vi "NI VeriStand - Open Workspace Tool.vi"(7 "Workspace Tool Path":path, 8 "error in (no error)":errorcluster, 11 "Project Ref in":T1) -> (0 "error out":errorcluster, 3 "Project Ref out":T1)   [LabVIEW 2020, in "NI_VS Project ExecutionAPI.lvlib"]
doc: "Opens a Workspace tool for an NI VeriStand project."
uses:
  <vilib>/NI VeriStand/Execution/Project/NI_VS Project ExecutionAPI.lvlib
  <vilib>/NI VeriStand/Execution/Project/Project Ref.ctl
  NationalInstruments.VeriStand.ClientAPI
  NationalInstruments.VeriStand
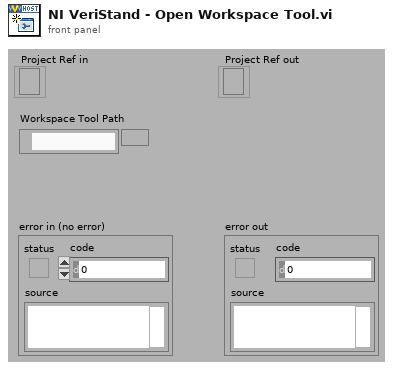
[diagram p1: front panel]
types:
  T1 = typedef "NI_VS Project ExecutionAPI.lvlib/Project Ref.ctl" = refnum<k24>
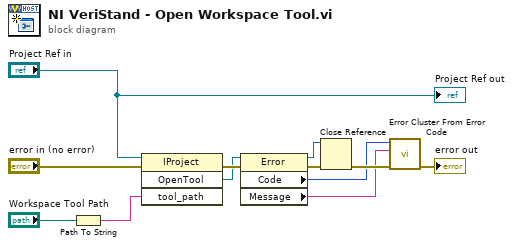
[diagram p0: block diagram]
diagram:
  n1 = Path To String(path="Workspace Tool Path") -> (string=w1:string)
  n2 = invoke class="IProject" method="OpenTool"(reference="Project Ref in", error in="error in (no error)", "tool_path"=w1) -> (error out=w10:errorcluster, "OpenTool"=w5:refnum<k24>)  [unwired: 1 in, 2 out]
  n3 = property class="Error"(reference=w5, error in=w10) -> (reference out=w8:refnum<k24>, error out=w9:errorcluster, "Code"=w4:u32, "Message"=w3:string)
  n4 = Close Reference(reference=w8, error in (no error)=w9) -> (error out=w7:errorcluster)
  n5 = call <vilib>:"Error Cluster From Error Code.vi"("error in (no error)"=w7, "error message (\"\")"=w3, "error code (0)"=w4) -> ("error out"=→"error out":errorcluster)  [unwired: 6 in]
  "Project Ref out" <- "Project Ref in"
